vi "configTestSeqLst.vi"(8 "error in (no error)":errorcluster, 11 "TestItemLst in":refnum<vi>) -> (0 "error out":errorcluster, 3 "TestItemLst out":refnum<vi>)   [LabVIEW 2010, in "pdbm_test_system.lvlib"]
uses:
  pdbm_test_system.lvlib
  <vilib>/picture/picture.llb/imagedata.ctl
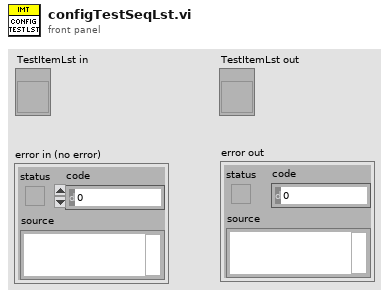
[diagram p1: front panel]
types:
  T1 = typedef "imagedata.ctl" = cluster{"image type":i32, "image depth":i32, "image":u8[], "mask":u8[], "colors":u32[], "Rectangle":cluster{"left":i16, "top":i16, "right":i16, "bottom":i16}}
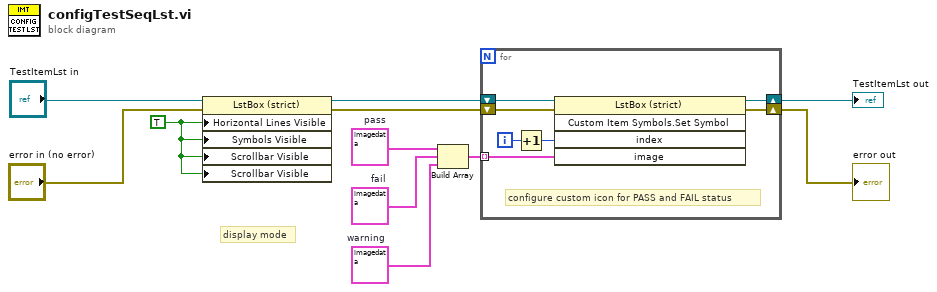
[diagram p0: block diagram]
diagram:
  w1 = T1 {"image type"=0, "image depth"=32, "image"=array[1024 elements], "mask"=[0, 0, 1, 128, 3, 192, 3, 192, 7, 224, 15, 240, 15, 240, 31, 248, 63, 252, 63, 252, 127, 254, 255, 255, 255, 255, 255, 255, 0, 0, 0, 0], "colors"=[], "Rectangle"={"left"=0, "top"=0, "right"=16, "bottom"=16}}  # warning
  w2 = T1 {"image type"=0, "image depth"=32, "image"=array[1024 elements], "mask"=[15, 224, 31, 240, 63, 248, 127, 252, 255, 254, 255, 254, 255, 254, 255, 254, 255, 254, 255, 254, 255, 254, 127, 252, 63, 248, 31, 240, 15, 224, 0, 0], "colors"=[], "Rectangle"={"left"=0, "top"=0, "right"=16, "bottom"=16}}  # fail
  w10 = T1 {"image type"=0, "image depth"=32, "image"=[0, 255, 255, 255, 0, 255, 255, 255, 0, 255, 255, 255, 0, 255, 255, 255, 0, 255, 255, 255, 0, 255, 255, 255, 0, 255, 255, 255, 0, 255, 255, 255, 0, 255, 255, 255, 0, 255, 255, 255, 0, 255, 255, 255, 0, 255, 255, 255, 0, 255, 255, 255, 0, 255, 255, 255, 0, 255, 255, 255, 0, 255, 255, 255, 0, 255, 255, 255, 0, 0, 0, 0, 0, 0, 0, 0, 0, 0, 0, 0, 51, 74, 140, 0, 187, 70, 137, 0, 255, 68, 135, 0, 255, 67, 135, 0, 255, 68, 135, 0, 255, 70, 137, 0, 187, 73, 139, 0, 51, 76, 141, 0, 0, 0, 0, 0, 0, 0, 0, 0, 0, 0, 0, 0, 0, 255, 255, 255, 0, 255, 255, 255, 0, 0, 0, 0, 0, 0, 0, 0, 149, 72, 138, 0, 255, 89, 150, 14, 255, 182, 213, 116, 255, 225, 244, 160, 255, 220, 239, 148, 255, 204, 230, 124, 255, 181, 214, 94, 255, 135, 181, 46, 255, 82, 145, 3, 170, 76, 140, 0, 0, 0, 0, 0, 0, 0, 0, 0, 0, 255, 255, 255, 0, 255, 255, 255, 0, 0, 0, 0, 170, 72, 138, 0, 255, 99, 156, 25, 255, 247, 255, 188, 255, 201, 228, 94, 255, 154, 197, 0, 255, 150, 195, 0, 255, 151, 196, 0, 255, 154, 197, 0, 255, 162, 202, 34, 255, 150, 193, 47, 255, 85, 147, 2, 149, 76, 141, 0, 0, 0, 0, 0, 0, 255, 255, 255, 0, 255, 255, 255, 51, 75, 140, 0, 255, 88, 148, 10, 255, 233, 248, 173, 255, 167, 208, 24, 255, 149, 196, 0, 255, 151, 198, 0, 255, 152, 198, 0, 255, 152, 199, 0, 255, 152, 199, 0, 255, 151, 198, 0, 255, 150, 197, 0, 255, 133, 181, 18, 255, 80, 143, 0, 51, 77, 142, 0, 0, 255, 255, 255, 0, 255, 255, 255, 190, 70, 136, 0, 255, 164, 201, 89, 255, 188, 222, 73, 255, 148, 199, 0, 255, 151, 200, 0, 255, 152, 201, 0, 255, 153, 201, 0, 255, 152, 201, 0, 255, 148, 199, 0, 255, 142, 195, 0, 255, 255, 255, 255, 255, 138, 189, 0, 255, 103, 160, 0, 191, 75, 139, 0, 0, 255, 255, 255, 0, 255, 255, 255, 255, 70, 136, 0, 255, 198, 224, 118, 255, 152, 203, 0, 255, 144, 197, 0, 255, 145, 198, 0, 255, 149, 200, 0, 255, 151, 201, 0, 255, 148, 200, 0, 255, 140, 195, 0, 255, 255, 255, 255, 255, 255, 255, 255, 255, 146, 199, 0, 255, 117, 171, 0, 255, 75, 140, 0, 0, 255, 255, 255, 0, 255, 255, 255, 255, 69, 136, 0, 255, 190, 221, 104, 255, 145, 201, 0, 255, 255, 255, 255, 255, 255, 255, 255, 255, 140, 198, 0, 255, 145, 200, 0, 255, 139, 197, 0, 255, 255, 255, 255, 255, 255, 255, 255, 255, 255, 255, 255, 255, 150, 204, 0, 255, 120, 173, 0, 255, 74, 139, 0, 0, 255, 255, 255, 0, 255, 255, 255, 255, 70, 137, 0, 255, 176, 210, 82, 255, 146, 204, 0, 255, 255, 255, 255, 255, 255, 255, 255, 255, 255, 255, 255, 255, 132, 196, 0, 255, 255, 255, 255, 255, 255, 255, 255, 255, 255, 255, 255, 255, 141, 200, 0, 255, 154, 208, 0, 255, 121, 173, 0, 255, 74, 139, 0, 0, 255, 255, 255, 0, 255, 255, 255, 255, 72, 138, 0, 255, 157, 196, 57, 255, 152, 209, 0, 255, 140, 203, 0, 255, 255, 255, 255, 255, 255, 255, 255, 255, 255, 255, 255, 255, 255, 255, 255, 255, 255, 255, 255, 255, 140, 202, 0, 255, 150, 207, 0, 255, 155, 210, 0, 255, 118, 171, 1, 255, 75, 140, 0, 0, 255, 255, 255, 0, 255, 255, 255, 201, 69, 131, 0, 255, 120, 171, 22, 255, 150, 201, 16, 255, 151, 211, 0, 255, 140, 205, 0, 255, 255, 255, 255, 255, 255, 255, 255, 255, 255, 255, 255, 255, 140, 204, 0, 255, 149, 209, 0, 255, 155, 213, 0, 255, 140, 193, 1, 255, 105, 161, 1, 201, 71, 132, 0, 0, 255, 255, 255, 0, 255, 255, 255, 81, 49, 89, 0, 255, 81, 144, 0, 255, 131, 180, 15, 255, 152, 210, 0, 255, 152, 213, 0, 255, 146, 209, 0, 255, 144, 207, 0, 255, 145, 208, 0, 255, 150, 211, 0, 255, 155, 214, 0, 255, 152, 209, 0, 255, 118, 171, 1, 255, 80, 144, 0, 81, 49, 90, 0, 0, 255, 255, 255, 0, 255, 255, 255, 10, 0, 0, 0, 170, 67, 124, 0, 255, 82, 145, 0, 255, 119, 172, 2, 255, 140, 195, 0, 255, 155, 215, 0, 255, 156, 218, 0, 255, 156, 218, 0, 255, 156, 215, 0, 255, 140, 195, 1, 255, 118, 171, 1, 255, 83, 146, 0, 170, 68, 124, 0, 10, 0, 0, 0, 0, 255, 255, 255, 0, 255, 255, 255, 0, 0, 0, 0, 30, 0, 0, 0, 187, 70, 128, 0, 255, 80, 144, 0, 255, 105, 161, 1, 255, 118, 171, 1, 255, 121, 172, 1, 255, 121, 172, 1, 255, 118, 171, 1, 255, 105, 161, 1, 255, 80, 144, 0, 170, 68, 124, 0, 30, 0, 0, 0, 0, 0, 0, 0, 0, 255, 255, 255, 0, 255, 255, 255, 0, 0, 0, 0, 0, 0, 0, 0, 34, 0, 0, 0, 92, 43, 79, 0, 201, 71, 131, 0, 255, 75, 140, 0, 255, 74, 139, 0, 255, 74, 139, 0, 255, 75, 140, 0, 201, 71, 131, 0, 92, 43, 79, 0, 30, 0, 0, 0, 0, 0, 0, 0, 0, 0, 0, 0, 0, 255, 255, 255, 0, 255, 255, 255, 0, 0, 0, 0, 0, 0, 0, 0, 0, 0, 0, 0, 10, 0, 0, 0, 37, 0, 0, 0, 51, 0, 0, 0, 51, 0, 0, 0, 51, 0, 0, 0, 51, 0, 0, 0, 37, 0, 0, 0, 10, 0, 0, 0, 0, 0, 0, 0, 0, 0, 0, 0, 0, 0, 0, 0, 0, 255, 255, 255], "mask"=[0, 0, 7, 224, 31, 248, 63, 252, 63, 252, 127, 254, 127, 254, 127, 254, 127, 254, 127, 254, 127, 254, 63, 252, 63, 252, 31, 248, 7, 224, 0, 0], "colors"=[], "Rectangle"={"left"=0, "top"=0, "right"=16, "bottom"=16}}  # pass
  w3 = TRUE ("Visible Items:Horizontal Lines Visible")
  # "display mode"
  n1 = property class="LstBox (strict)"(reference="TestItemLst in", error in="error in (no error)", "Horizontal Lines Visible"=w3, "Symbols Visible"=w3, "Scrollbar Visible"=w3, "Scrollbar Visible"=w3) -> (reference out=w9:refnum<vi>, error out=w8:errorcluster)
  n2 = Build Array(w10, w2, w1) -> (w7:T1[])
  n3 = for {
    shift-right: [w17] -> w4
    shift-left: w9 -> [w18]
    shift-right: [w12] -> w6
    shift-left: w8 -> [w16]
    tunnel: w7 -> [w13] mode=indexing
    i -> [w15]
    # "configure custom icon for PASS and FAIL status"
    n4 = Increment(x=w15) -> (x+1=w14:i32)
    n5 = invoke class="LstBox (strict)" method="Custom Item Symbols.Set Symbol"(reference=w18, error in=w16, "index"=w14, "image"=w13) -> (reference out=w17:refnum<vi>, error out=w12:errorcluster)  [unwired: 1 in, 3 out]
  }
  "error out" <- w6
  "TestItemLst out" <- w4
